vi "OpenConnectionToServer.vi"(4 "port":u16=6341, 5 "machine":string="localhost") -> (0 "error out":errorcluster, 2 "TCP Network Connection Refnum":refnum<k5>)   [LabVIEW 2011]
doc: "And the description is..."
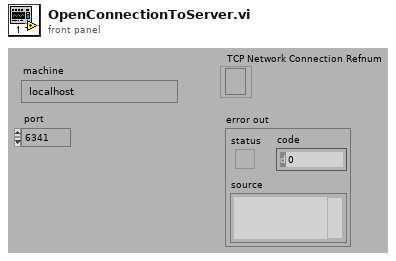
[diagram p1: front panel]
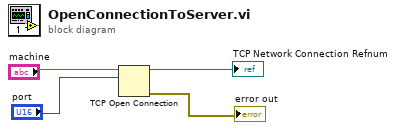
[diagram p0: block diagram]
diagram:
  n1 = TCP Open Connection(address="machine", remote port or service name="port") -> (connection ID=→"TCP Network Connection Refnum":refnum<k5>, error out=→"error out":errorcluster)  [unwired: 1 in, 2 out]
